vi "Delete Private Data.vi"(8 "error in (no error)":errorcluster, 11 "LVClassLibrary in":refnum<vi>) -> (0 "error out":errorcluster)   [LabVIEW 2020, in "Message Rescripter.lvlib"]
uses:
  Message Rescripter.lvlib
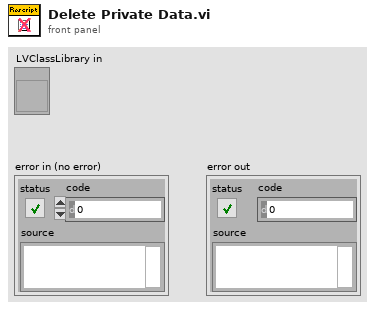
[diagram p1: front panel]
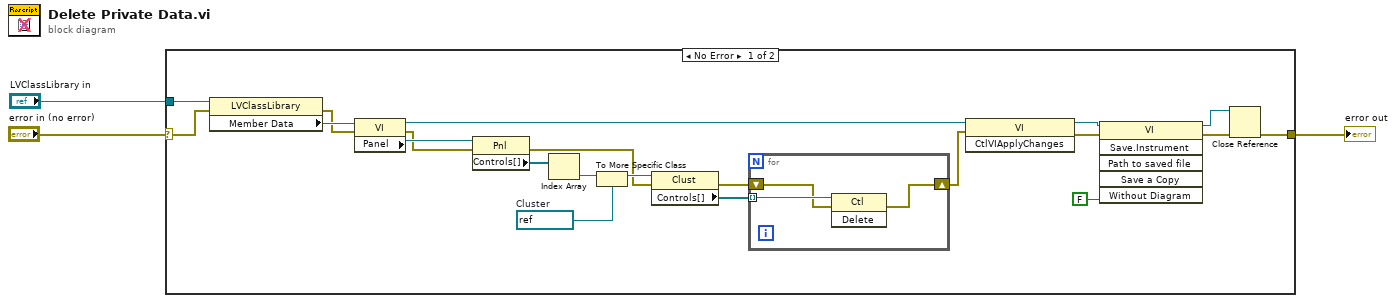
[diagram p0: block diagram]
diagram:
  n1 = case shown="No Error" "error in (no error)" {
    selector: "error in (no error)" -> [w4 w28]
    tunnel: "LVClassLibrary in" -> [w22 _]
    tunnel: [w9 w28] -> w2
    frame No Error {
      w19 = refnum<vi> refnum  # Cluster
      n2 = property class="LVClassLibrary"(reference=w22, error in=w4) -> (error out=w5:errorcluster, "Member Data"=w8:refnum<vi>)  [unwired: 1 out]
      n3 = property class="VI"(reference=w8, error in=w5) -> (reference out=w11:refnum<vi>, error out=w12:errorcluster, "Panel"=w23:refnum<vi>)
      n4 = property class="Pnl"(reference=w23, error in=w12) -> (error out=w18:errorcluster, "Controls[]"=w24:refnum<vi>[])  [unwired: 1 out]
      n5 = Index Array(array=w24) -> (element=w21:refnum<vi>)  [unwired: 1 in]
      n6 = To More Specific Class(target class=w19, reference=w21) -> (specific class reference=w20:refnum<vi>)  [unwired: 1 in, 1 out]
      n7 = property class="Clust"(reference=w20, error in=w18) -> (error out=w17:errorcluster, "Controls[]"=w16:refnum<vi>[])  [unwired: 1 out]
      n8 = for {
        tunnel: w16 -> [w27] mode=indexing
        shift-right: [w25] -> w10
        shift-left: w17 -> [w26]
        n9 = invoke class="Ctl" method="Delete"(reference=w27, error in=w26) -> (error out=w25:errorcluster)  [unwired: 1 in, 2 out]
      }
      n10 = invoke class="VI" method="CtlVIApplyChanges"(reference=w11, error in=w10) -> (reference out=w13:refnum<vi>, error out=w14:errorcluster)  [unwired: 1 in, 1 out]
      n11 = invoke class="VI" method="Save.Instrument"(reference=w13, error in=w14, "Save a Copy"=FALSE) -> (reference out=w7:refnum<vi>, error out=w6:errorcluster)  [unwired: 3 in, 4 out]
      n12 = Close Reference(reference=w7, error in (no error)=w6) -> (error out=w9:errorcluster)
    }
    frame Error {
    }
  }
  "error out" <- w2
